vi "Get Test Methods.vi"(8 "error in (no error)":errorcluster, 11 "Parameterized Test Case in":refnum<class "Parameterized Test Case.lvclass">) -> (0 "error out":errorcluster, 2 "Array":path[](array[path]), 3 "Parameterized Test Case out":refnum<class "Parameterized Test Case.lvclass">)   [LabVIEW 2020, in "Parameter.lvclass"]
uses:
  Parameter.lvclass
  Parameterized Test Case/Parameterized Test Case.lvclass
  Parameter.lvclass/Parameter.ctl
  <resource>/objmgr/DOMUserDefRef.rc
  <vilib>/xml/NI_XML.lvlib
  <vilib>/xml/Close Reference(Node).vi
  C:/Program Files (x86)/National Instruments/LabVIEW 2020/vi.lib/Astemes/LUnit/Test Case.lvclass
  C:/Program Files (x86)/National Instruments/LabVIEW 2020/vi.lib/Astemes/LUnit/LUnit Runnable.lvclass
  C:/git/astemes-lunit-parameterized-test/source/Parameterized Test Case/Parameterized Test Case.lvclass
  <vilib>/xml/Load XML File.vi
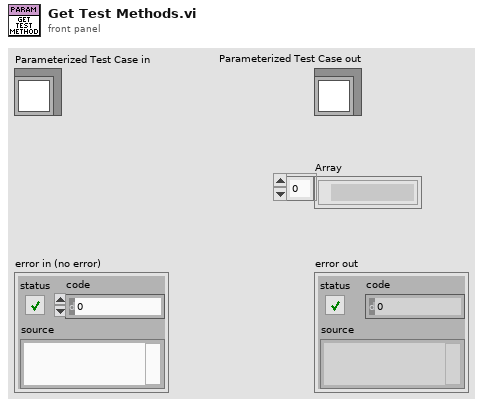
[diagram p1: front panel]
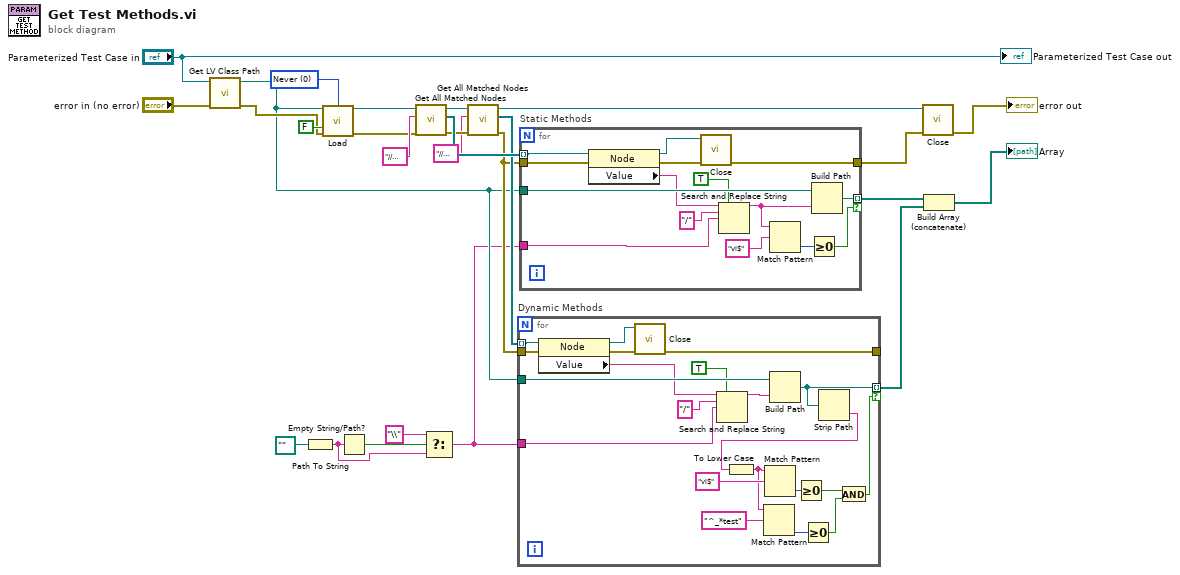
[diagram p0: block diagram]
diagram:
  w26 = 0 items=["Never", "Always", "Auto"] ("validate on load (Auto)")
  n1 = call <vilib>:"Get LV Class Path.vi"("error in (no error)"="error in (no error)", "object"="Parameterized Test Case in") -> ("error out"=w18:errorcluster, "class path"=w11:path)  [unwired: 8 in]
  n2 = Path To String(path=path "") -> (string=w6:string)
  n3 = call-poly <vilib>:"Load.vi"("path to XML document"=w11, "validate on load (Auto)"=w26, "load external DTD (True)"=FALSE, "error in (no error)"=w18) -> ("DOM document out"=w24:refnum<k20>, "error out"=w20:errorcluster)  [unwired: 9 in, 1 out]
  n4 = Empty String/Path?(string/path=w6) -> (empty?=w8:bool)
  n5 = call <vilib>:"Get All Matched Nodes.vi"("error in (no error)"=w20, "XPath expression"="//Item[@Type='VI'][Property[@Name='NI.ClassItem.InvokeUsage']='0'\n    or Property[@Name='NI.ClassItem.IsStaticMethod']='true'][Property[@Name='NI.ClassItem.MethodScope']='1']/@URL", "node in"=w24) -> ("error out"=w15:errorcluster, "node result array"=w22:refnum<k20>[], "node out"=w17:refnum<k20>)  [unwired: 6 out]
  n6 = Select(t="\\" ("search string"), s=w8, f=w6) -> (s? t:f=w5:string)
  n7 = call <vilib>:"Get All Matched Nodes.vi"("error in (no error)"=w15, "XPath expression"="//Item[@Type='VI'][Property[@Name='NI.ClassItem.InvokeUsage']='1'\n    or Property[@Name='NI.ClassItem.IsStaticMethod']='false'][Property[@Name='NI.ClassItem.MethodScope']='1']/@URL", "node in"=w17) -> ("error out"=w12:errorcluster, "node result array"=w13:refnum<k20>[], "node out"=w16:refnum<k20>)  [unwired: 6 out]
  n8 = for "Dynamic Methods" {
    tunnel: w13 -> [w47] mode=indexing
    tunnel: w12 -> [w46]
    tunnel: [w43] -> _
    tunnel: w11 -> [w41]
    tunnel: [w31] -> w10 mode=indexing if=w32
    tunnel: w5 -> [w27]
    n9 = property class="Node"(reference=w47, error in=w46) -> (reference out=w45:refnum<k20>, error out=w44:errorcluster, "Value"=w40:string)
    n10 = call-poly <vilib>:"Close.vi"("error in (no error)"=w44, "node"=w45) -> ("error out"=w43:errorcluster)  [unwired: 7 out]
    n11 = Search and Replace String(replace all?=TRUE ("replace all? (F)"), input string=w40, search string="/", replace string=w27) -> (result string=w30:string)  [unwired: 4 in, 3 out]
    n12 = Build Path(base path=w41, name or relative path=w30) -> (appended path=w31:path)
    n13 = Strip Path(path=w31) -> (name=w29:string)  [unwired: 1 out]
    n14 = To Lower Case(string=w29) -> (all lower case string=w28:string)
    n15 = Match Pattern(string=w28, regular expression="^_*test") -> (offset past match=w36:i32)  [unwired: 1 in, 3 out]
    n16 = Match Pattern(string=w28, regular expression="vi$") -> (offset past match=w38:i32)  [unwired: 1 in, 3 out]
    n17 = Greater Or Equal To 0?(x=w38) -> (x >= 0?=w33:bool)
    n18 = Greater Or Equal To 0?(x=w36) -> (x >= 0?=w34:bool)
    n19 = And(x=w33, y=w34) -> (x .and. y?=w32:bool)
  }
  n20 = for "Static Methods" {
    tunnel: w22 -> [w62] mode=indexing
    tunnel: w12 -> [w61]
    tunnel: [w58] -> w21
    tunnel: w11 -> [w56]
    tunnel: [w55] -> w19 mode=indexing if=w51
    tunnel: w5 -> [w48]
    n21 = property class="Node"(reference=w62, error in=w61) -> (reference out=w60:refnum<k20>, error out=w59:errorcluster, "Value"=w54:string)
    n22 = call-poly <vilib>:"Close.vi"("error in (no error)"=w59, "node"=w60) -> ("error out"=w58:errorcluster)  [unwired: 7 out]
    n23 = Search and Replace String(replace all?=TRUE ("replace all? (F)"), input string=w54, search string="/", replace string=w48) -> (result string=w50:string)  [unwired: 4 in, 3 out]
    n24 = Match Pattern(string=w50, regular expression="vi$") -> (offset past match=w52:i32)  [unwired: 1 in, 3 out]
    n25 = Greater Or Equal To 0?(x=w52) -> (x >= 0?=w51:bool)
    n26 = Build Path(base path=w56, name or relative path=w50) -> (appended path=w55:path)
  }
  n27 = call-poly <vilib>:"Close.vi"("error in (no error)"=w21, "node"=w16) -> ("error out"=→"error out":errorcluster)  [unwired: 7 out]
  n28 = Build Array (concatenate)(w19, w10) -> (→"Array":path[])
  "Parameterized Test Case out" <- "Parameterized Test Case in"
